vi "Table Buffer - Check.vi"(8 "error in (no error)":errorcluster) -> (0 "error out":errorcluster, 2 "Buffer Full":bool, 3 "# Elements in Buffer":i32)   [LabVIEW 2025, in "I2C Bus Monitor UI.lvlib"]
uses:
  I2C Bus Monitor UI.lvlib
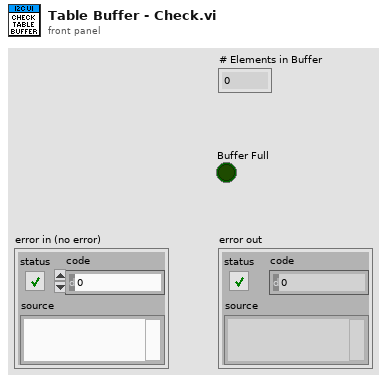
[diagram p1: front panel]
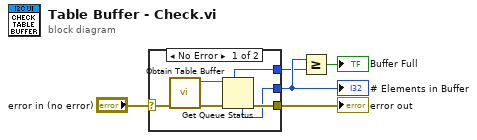
[diagram p0: block diagram]
diagram:
  n1 = case shown="No Error" "error in (no error)" {
    selector: "error in (no error)" -> [w11 w12]
    tunnel: [w9 w12] -> w4
    tunnel: [w7 _] -> w3
    tunnel: [w6 _] -> w2
    frame No Error {
      n2 = call "Obtain Table Buffer.vi"("error in (no error)"=w11) -> ("error out"=w10:errorcluster, "Table Queue"=w8:refnum<queue>)  [unwired: 9 in]
      n3 = Get Queue Status(queue=w8, error in (no error)=w10) -> (max queue size=w6:i32, error out=w9:errorcluster, # elements in queue=w7:i32)  [unwired: 1 in, 5 out]
    }
    frame Error {
    }
  }
  "error out" <- w4
  "# Elements in Buffer" <- w3
  n4 = Greater Or Equal?(x=w3, y=w2) -> (x >= y?=→"Buffer Full":bool)
